vi "Spectrum_analyzer.vi"() -> ()   [LabVIEW 2024]
uses:
  <vilib>/Utility/file.llb/Write Delimited Spreadsheet (DBL).vi
  Downloads/agilent_esa_psa_series/Agilent ESA PSA Series/Agilent ESA PSA Series.lvlib
panel:
  out "Data Graph":T1(graph)
  in  "file path (dialog if empty)":path=path "C:/Users/hamza/OneDrive/Desktop/study/bbb.txt"
  in  "error in (no error)":errorcluster
  in  "VISA resource name":refnum<visa-resource-name>="GPIB0::18::INSTR"
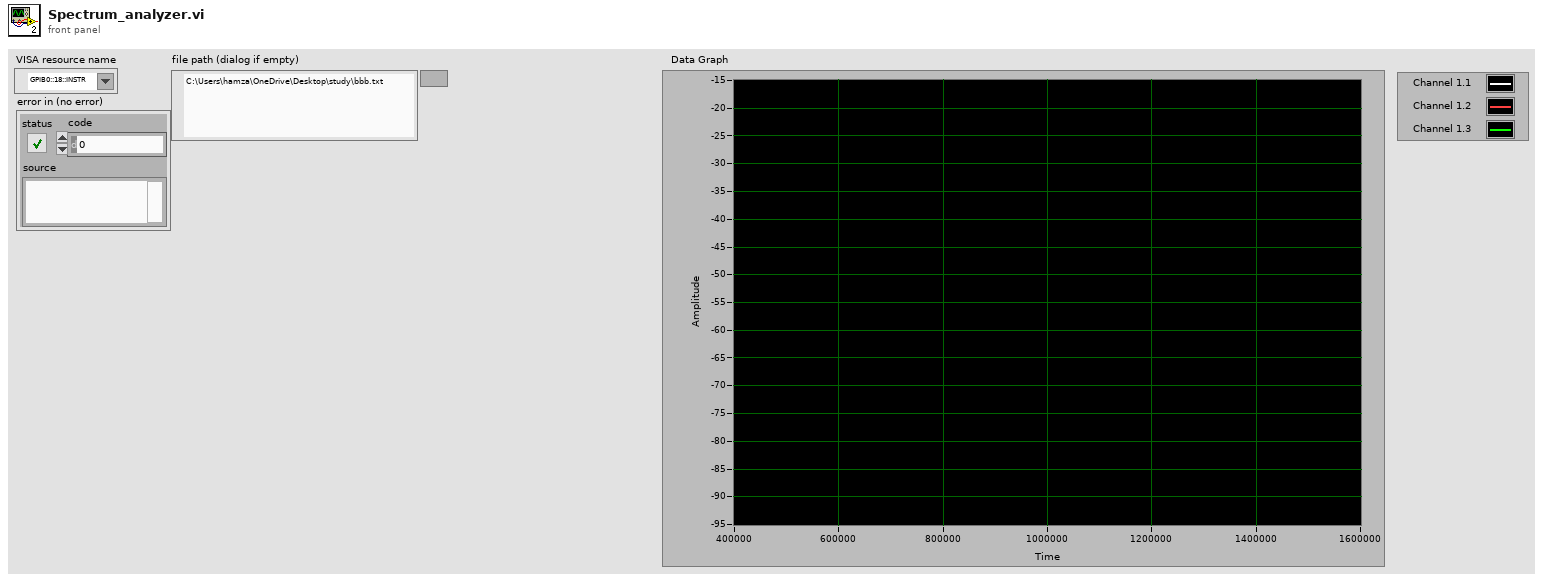
[diagram p1: front panel]
types:
  T1 = cluster{"Initial X":dbl, "X Increment":dbl, "Trace Array":dbl[]}[]
  T2 = cluster{"Initial X":dbl, "X Increment":dbl, "Trace Array":dbl[]}
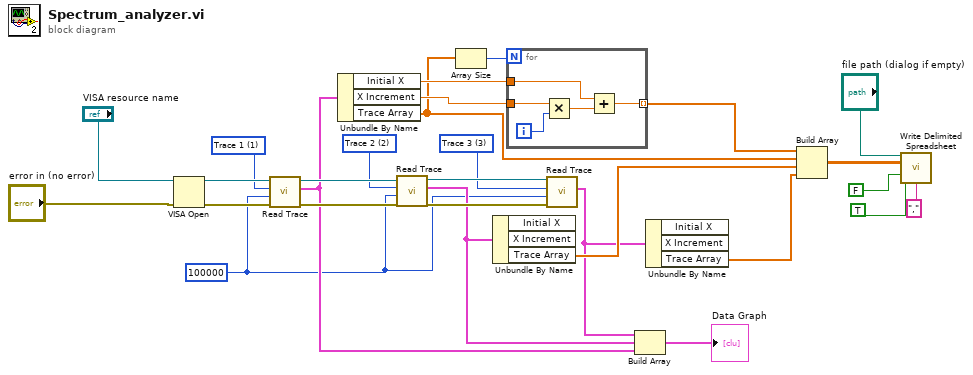
[diagram p0: block diagram]
diagram:
  w1 = 100000 ("Maximum Time (10000 ms)")
  w16 = u16 3 items=["Trace 1"=1, "Trace 2"=2, "Trace 3"=3] ("Trace Name (1: Trace 1)")
  w18 = u16 2 items=["Trace 1"=1, "Trace 2"=2, "Trace 3"=3] ("Trace Name (1: Trace 1)")
  w25 = u16 1 items=["Trace 1"=1, "Trace 2"=2, "Trace 3"=3] ("Trace Name (1: Trace 1)")
  n1 = VISA Open(error in (no error)="error in (no error)", VISA resource name="VISA resource name") -> (VISA resource name=w26:refnum<visa-resource-name>, error out=w24:errorcluster)  [unwired: 3 in]
  n2 = call "Read Trace.vi"("error in (no error)"=w24, "Maximum Time (10000 ms)"=w1, "Trace Name (1: Trace 1)"=w25, "VISA resource name"=w26) -> ("error out"=w19:errorcluster, "Trace Waveform"=w4:T2, "VISA resource name out"=w20:refnum<visa-resource-name>)  [unwired: 5 in]
  n3 = Unbundle By Name(w4) -> ("Initial X"=w21:dbl, "X Increment"=w22:dbl, "Trace Array"=w13:dbl[])
  n4 = call "Read Trace.vi"("error in (no error)"=w19, "Maximum Time (10000 ms)"=w1, "Trace Name (1: Trace 1)"=w18, "VISA resource name"=w20) -> ("error out"=w15:errorcluster, "Trace Waveform"=w3:T2, "VISA resource name out"=w17:refnum<visa-resource-name>)  [unwired: 5 in]
  n5 = Array Size(array=w13) -> (size(s)=w23:i32)
  n6 = Unbundle By Name(w3) -> ("Trace Array"=w12:dbl[])  [unwired: 2 out]
  n7 = for {
    N: w23 -> [_]
    tunnel: w22 -> [w31]
    tunnel: w21 -> [w30]
    tunnel: [w33] -> w14 mode=indexing
    i -> [w32]
    n8 = Multiply(x=w31, y=w32) -> (x*y=w29:dbl)
    n9 = Add(x=w30, y=w29) -> (x+y=w33:dbl)
  }
  n10 = call "Read Trace.vi"("error in (no error)"=w15, "Maximum Time (10000 ms)"=w1, "Trace Name (1: Trace 1)"=w16, "VISA resource name"=w17) -> ("Trace Waveform"=w5:T2)  [unwired: 5 in, 2 out]
  n11 = Build Array(w5, w3, w4) -> (→"Data Graph":T1)
  n12 = Unbundle By Name(w5) -> ("Trace Array"=w11:dbl[])  [unwired: 2 out]
  n13 = Build Array(w14, w13, w12, w11) -> (w10:dbl[][])
  n14 = call-poly <vilib>:"Write Delimited Spreadsheet.vi"("file path (dialog if empty)"="file path (dialog if empty)", "2D data"=w10, "append to file? (new file:F)"=FALSE, "transpose? (no:F)"=TRUE, "delimiter (\\t)"="," ("delimiter (\\t)")) -> ()  [unwired: 9 in, 2 out]
